vi "Design_Yiran.vi"() -> ()   [LabVIEW 2025]
panel:
  out "Initial height3":dbl[](array[numeric])
  out "Initial height 2":dbl[](array[numeric])
  in  "Initial Velocity-y":dbl
  in  "Initial height":dbl[](array[numeric])
  in  "Initial Velocity - x":dbl
  in  "Mass":dbl
  out "XY Graph":cluster{"X":dbl, "Y":dbl}[](graph)
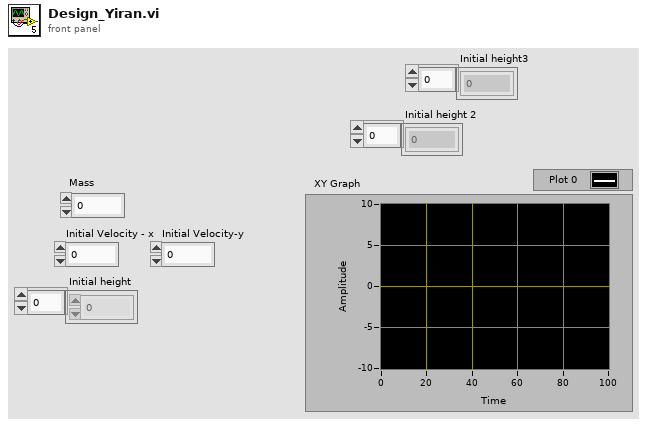
[diagram p1: front panel]
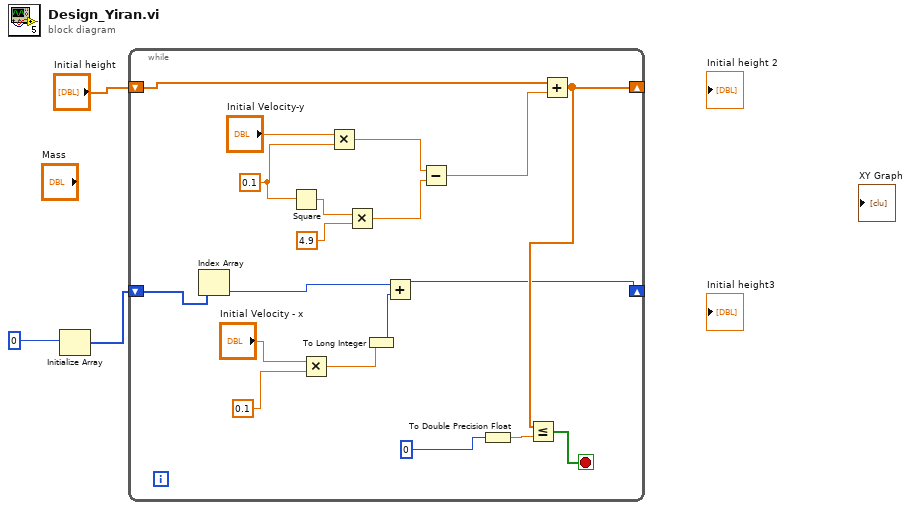
[diagram p0: block diagram]
diagram:
  n1 = Initialize Array(0) -> (w1:i32[])  [unwired: 1 in]
  n2 = while {
    shift-right: [w10] -> _
    shift-left: "Initial height" -> [w14]
    shift-right: [w5] -> w4
    shift-left: w1 -> [w8]
    stop <- w22 stop-if-true
    w20 = 0.1
    n3 = Index Array(array=w8) -> (element=w7:i32)  [unwired: 1 in]
    n4 = Square(x=w20) -> (x^2=w19:dbl)
    n5 = Multiply(x="Initial Velocity - x", y=0.1) -> (x*y=w11:dbl)
    n6 = Multiply(x="Initial Velocity-y", y=w20) -> (x*y=w17:dbl)
    n7 = Multiply(x=w19, y=4.9) -> (x*y=w16:dbl)
    n8 = To Long Integer(number=w11) -> (32bit integer=w6:i32)
    n9 = Add(x=w7, y=w6) -> (x+y=w5:i32)
    n10 = Subtract(x=w17, y=w16) -> (x-y=w15:dbl)
    n11 = To Double Precision Float(number=0) -> (double precision float=w9:dbl)
    n12 = Add(x=w14, y=w15) -> (x+y=w10:dbl[])
    n13 = Less Or Equal?(x=w10, y=w9) -> (x <= y?=w22:bool[])
  }
